vi "Remove_Legend3.vi"(1 "Ordinate Strings":string[](array[string])) -> (0 "Array":string[](array[string]))   [LabVIEW 2020]
uses:
  <vilib>/Utility/error.llb/whitespace.ctl
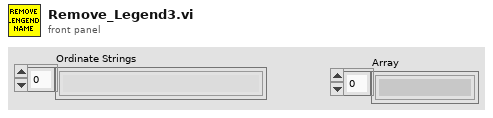
[diagram p1: front panel]
types:
  T1 = typedef "whitespace.ctl" = u16
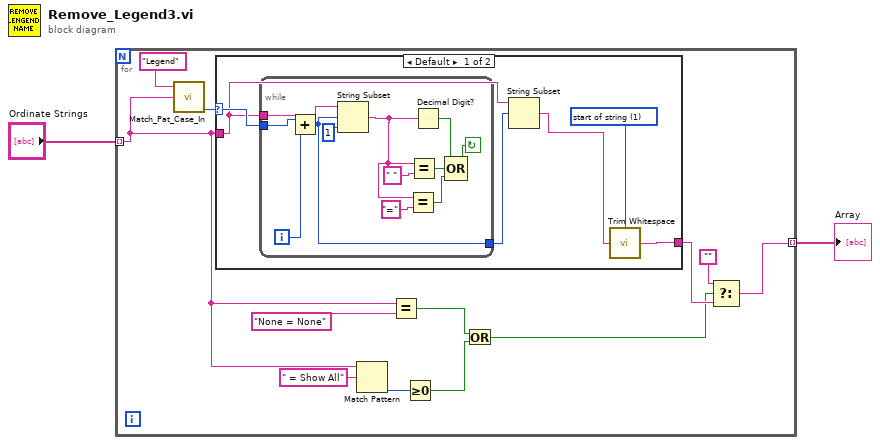
[diagram p0: block diagram]
diagram:
  n1 = for {
    tunnel: "Ordinate Strings" -> [w8] mode=indexing
    tunnel: [w10] -> w2 mode=indexing
    n2 = call "Match_Pat_Case_In.vi"("String to match"="Legend", "String"=w8) -> ("offset past match"=w13:i32)  [unwired: 1 in, 3 out]
    n3 = case shown="Default" w13 {
      selector: w13 -> [w20 _]
      tunnel: w8 -> [w15 w33]
      tunnel: [w18 w33] -> w11
      frame Default {
        w19 = T1 1 items=["both", "start of string", "end of string"] ("location (both)")
        n4 = while {
          tunnel: w20 -> [w30]
          tunnel: w15 -> [w32]
          tunnel: [w28] -> w17
          i -> [w29]
          stop <- w21 continue-if-true
          n5 = Add(x=w30, y=w29) -> (x+y=w28:i32)
          n6 = String Subset(string=w32, offset (0)=w28, length (rest)=1 ("length (rest)")) -> (substring=w23:string)
          n7 = Equal?(x=w23, y="=") -> (x = y?=w26:bool)
          n8 = Equal?(x=w23, y=" ") -> (x = y?=w27:bool)
          n9 = Decimal Digit?(1:w23) -> (0:w22:bool)
          n10 = Compound Arithmetic op=OR(w22, w27, w26) -> (w21:bool)
        }
        n11 = String Subset(string=w15, offset (0)=w17) -> (substring=w16:string)  [unwired: 1 in]
        n12 = call <vilib>:"Trim Whitespace.vi"("string"=w16, "location (both)"=w19) -> ("trimmed string"=w18:string)
      }
      frame -1 {
      }
    }
    n13 = Match Pattern(string=w8, regular expression=" = Show All") -> (offset past match=w6:i32)  [unwired: 1 in, 3 out]
    n14 = Equal?(x=w8, y="None = None") -> (x = y?=w4:bool)
    n15 = Greater Or Equal To 0?(x=w6) -> (x >= 0?=w5:bool)
    n16 = Or(x=w4, y=w5) -> (x .or. y?=w3:bool)
    n17 = Select(t="", s=w3, f=w11) -> (s? t:f=w10:string)
  }
  "Array" <- w2
